vi "Bring Caller to Front.vi"(8 "Error In":errorcluster) -> (0 "Error Out":errorcluster)   [LabVIEW 2014]
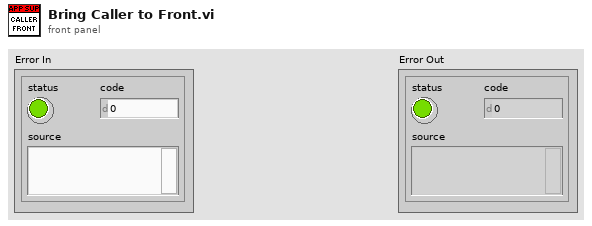
[diagram p1: front panel]
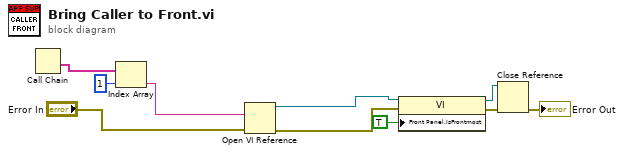
[diagram p0: block diagram]
diagram:
  n1 = Call Chain() -> (call chain=w6:string[])
  n2 = Index Array(array=w6, index=1) -> (element=w4:string)
  n3 = Open VI Reference(vi path=w4, error in (no error)="Error In") -> (vi reference=w1:refnum<vi>, error out=w2:errorcluster)  [unwired: 4 in]
  n4 = property class="VI"(reference=w1, error in=w2, "Front Panel.IsFrontmost"=TRUE ("Front Panel Window:Is Frontmost")) -> (reference out=w9:refnum<vi>, error out=w8:errorcluster)
  n5 = Close Reference(reference=w9, error in (no error)=w8) -> (error out=→"Error Out":errorcluster)
